vi "8-bit video exporter window menu.vi"(8 "error in (no error)":errorcluster, 11 "menu":refnum<k9>) -> (0 "error out":errorcluster, 3 "menu reference out":refnum<k9>)   [LabVIEW 2013]
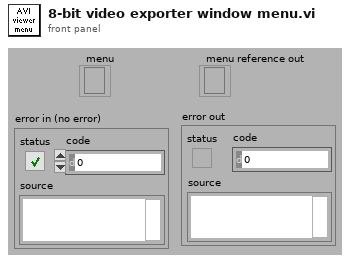
[diagram p1: front panel]
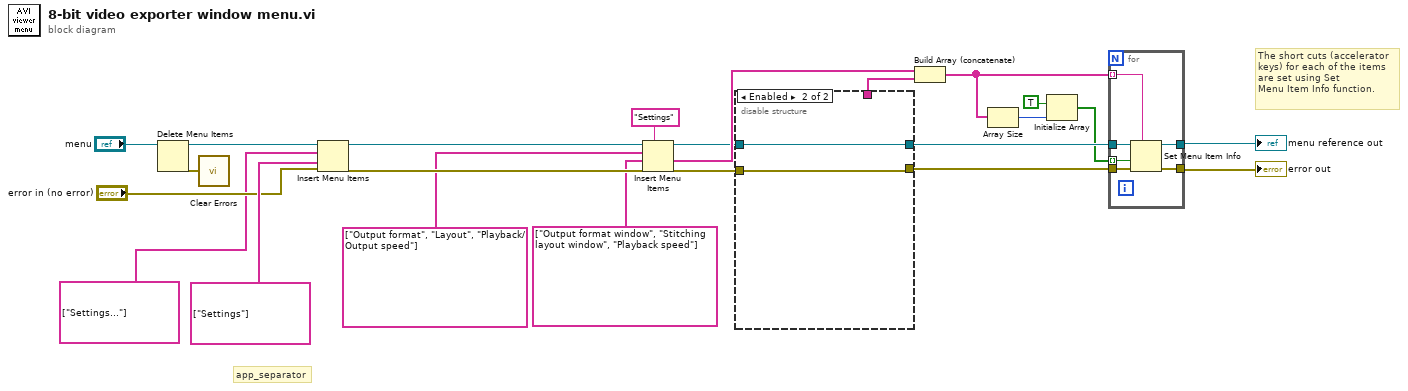
[diagram p0: block diagram]
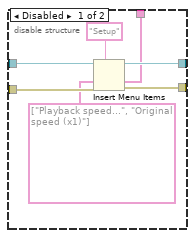
[diagram p2: hidden frame]
diagram:
  # "app_separator"
  # "The short cuts (accelerator\nkeys) for each of the items\nare set using Set\nMenu Item Info function."
  n1 = Delete Menu Items(9:"menu") -> (0:w17:errorcluster, 3:w20:refnum<k9>)  [unwired: 2 in, 1 out]
  n2 = call <vilib>:"Clear Errors.vi"("error in (no error)"=w17) -> ()  [unwired: 6 in, 1 out]
  n3 = Insert Menu Items(6:"error in (no error)", 7:string[] ["Settings"] ("item tags"), 8:string[] ["Settings..."] ("item tags"), 9:w20) -> (0:w22:errorcluster, 3:w18:refnum<k9>)  [unwired: 3 out]
  n4 = Insert Menu Items(5:"Settings" ("menu tag"), 6:w22, 7:string[] ["Output format window", "Stitching layout window", "Playback speed"] ("item tags"), 8:string[] ["Output format", "Layout", "Playback/Output speed"] ("item tags"), 9:w18) -> (0:w13:errorcluster, 1:w12:string[], 3:w10:refnum<k9>)  [unwired: 1 out]
  n5 = disable-structure shown="Enabled" {
    disable-tunnel: w13 -> [w30 w31]
    disable-tunnel: w10 -> [w29 w32]
    disable-tunnel: [w28 w31] -> w9
    disable-tunnel: [w27 w32] -> w8
    disable-tunnel: [w26 _] -> w7
    frame Disabled {
      n6 = Insert Menu Items(5:"Setup" ("menu tag"), 6:w30, 7:string[] ["Playback speed...", "Original speed (x1)"] ("item tags"), 9:w29) -> (0:w28:errorcluster, 1:w26:string[], 3:w27:refnum<k9>)  [unwired: 2 out]
    }
    frame Enabled {
    }
  }
  n7 = Build Array (concatenate)(w12, w7) -> (w4:string[])
  n8 = Array Size(array=w4) -> (size(s)=w6:i32)
  n9 = Initialize Array(TRUE, w6) -> (w5:bool[])
  n10 = for {
    tunnel: w8 -> [w38]
    tunnel: [w37] -> w19
    tunnel: w4 -> [w36] mode=indexing
    tunnel: w9 -> [w35]
    tunnel: [w34] -> w23
    tunnel: w5 -> [w33] mode=indexing
    n11 = Set Menu Item Info(7:w36, 8:w35, 9:w33, 11:w38) -> (0:w34:errorcluster, 3:w37:refnum<k9>)  [unwired: 1 in, 2 out]
  }
  "error out" <- w23
  "menu reference out" <- w19
